vi "Lab_3.vi"() -> ()   [LabVIEW 2021]
panel:
  out "Real":dbl
  in  "Set_point":dbl
  out "k1":dbl[][](array[numeric])
  out "L":dbl[](array[numeric])
  out "p2":cdb
  out "p1":cdb
  out "p2_o":cdb
  out "p1_o":cdb
  in  "tso":dbl
  out "ks":dbl[][](array[numeric])
  out "Ki":dbl[][](array[numeric])
  out "K":dbl[](array[numeric])
  in  "T":dbl
  in  "tss":dbl
  in  "Fa":dbl
  in  "Orden":dbl
  out "Controlable":string="El sistema es Observable"
  out "Observable":string="El sistema es Observable"
  out "Waveform Chart 2":dbl[][](graph)
  out "Waveform Chart":dbl[][](graph)
  out "det_Mc":dbl
  out "det_Mo":dbl
  out "B_O":dbl[][](array[numeric])
  out "C_O":dbl[][](array[numeric])
  out "A_O":dbl[][](array[numeric])
  out "Rango_Con":dbl
  out "Rango_Obs":dbl
  out "C":dbl[][](array[numeric])
  out "B":dbl[][](array[numeric])
  out "A":dbl[][](array[numeric])
  out "Mo":dbl[][](array[numeric])
  out "Mc":dbl[][](array[numeric])
  in  "b4":dbl
  in  "b3":dbl
  in  "b2":dbl
  in  "b1":dbl
  in  "a4":dbl
  in  "a3":dbl
  in  "a2":dbl
  in  "a1":dbl
  # "Forma canónica observable (FCO)"
  # "Forma canónica controlable (FCC)"
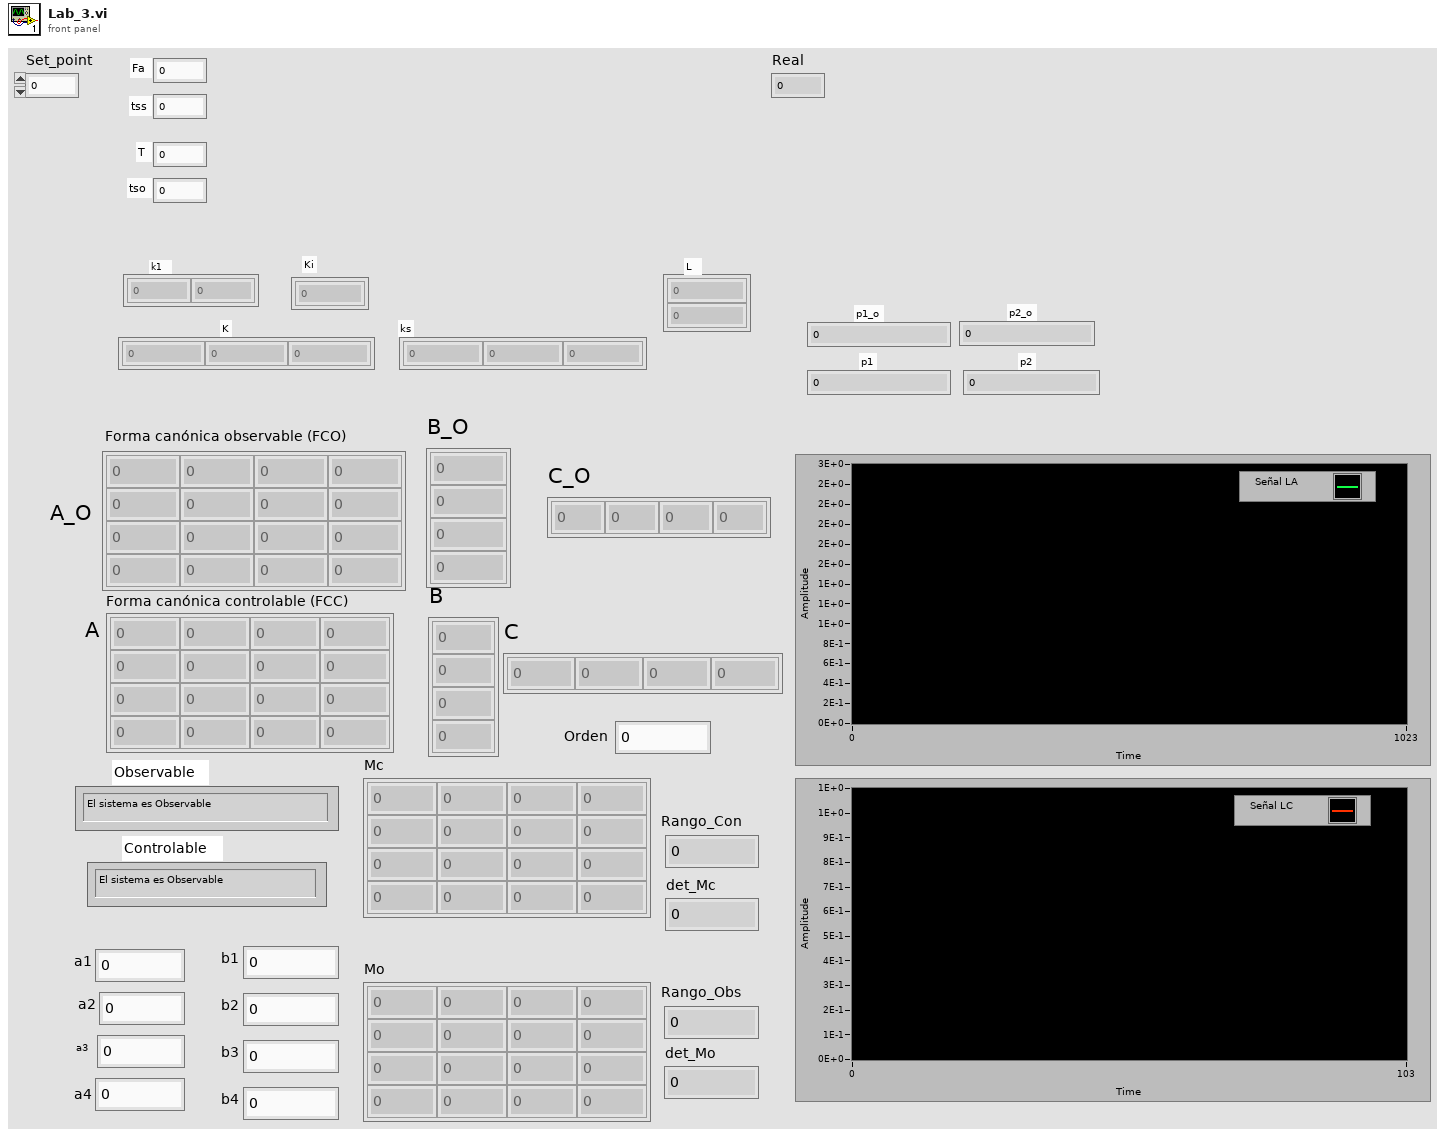
[diagram p1: front panel]
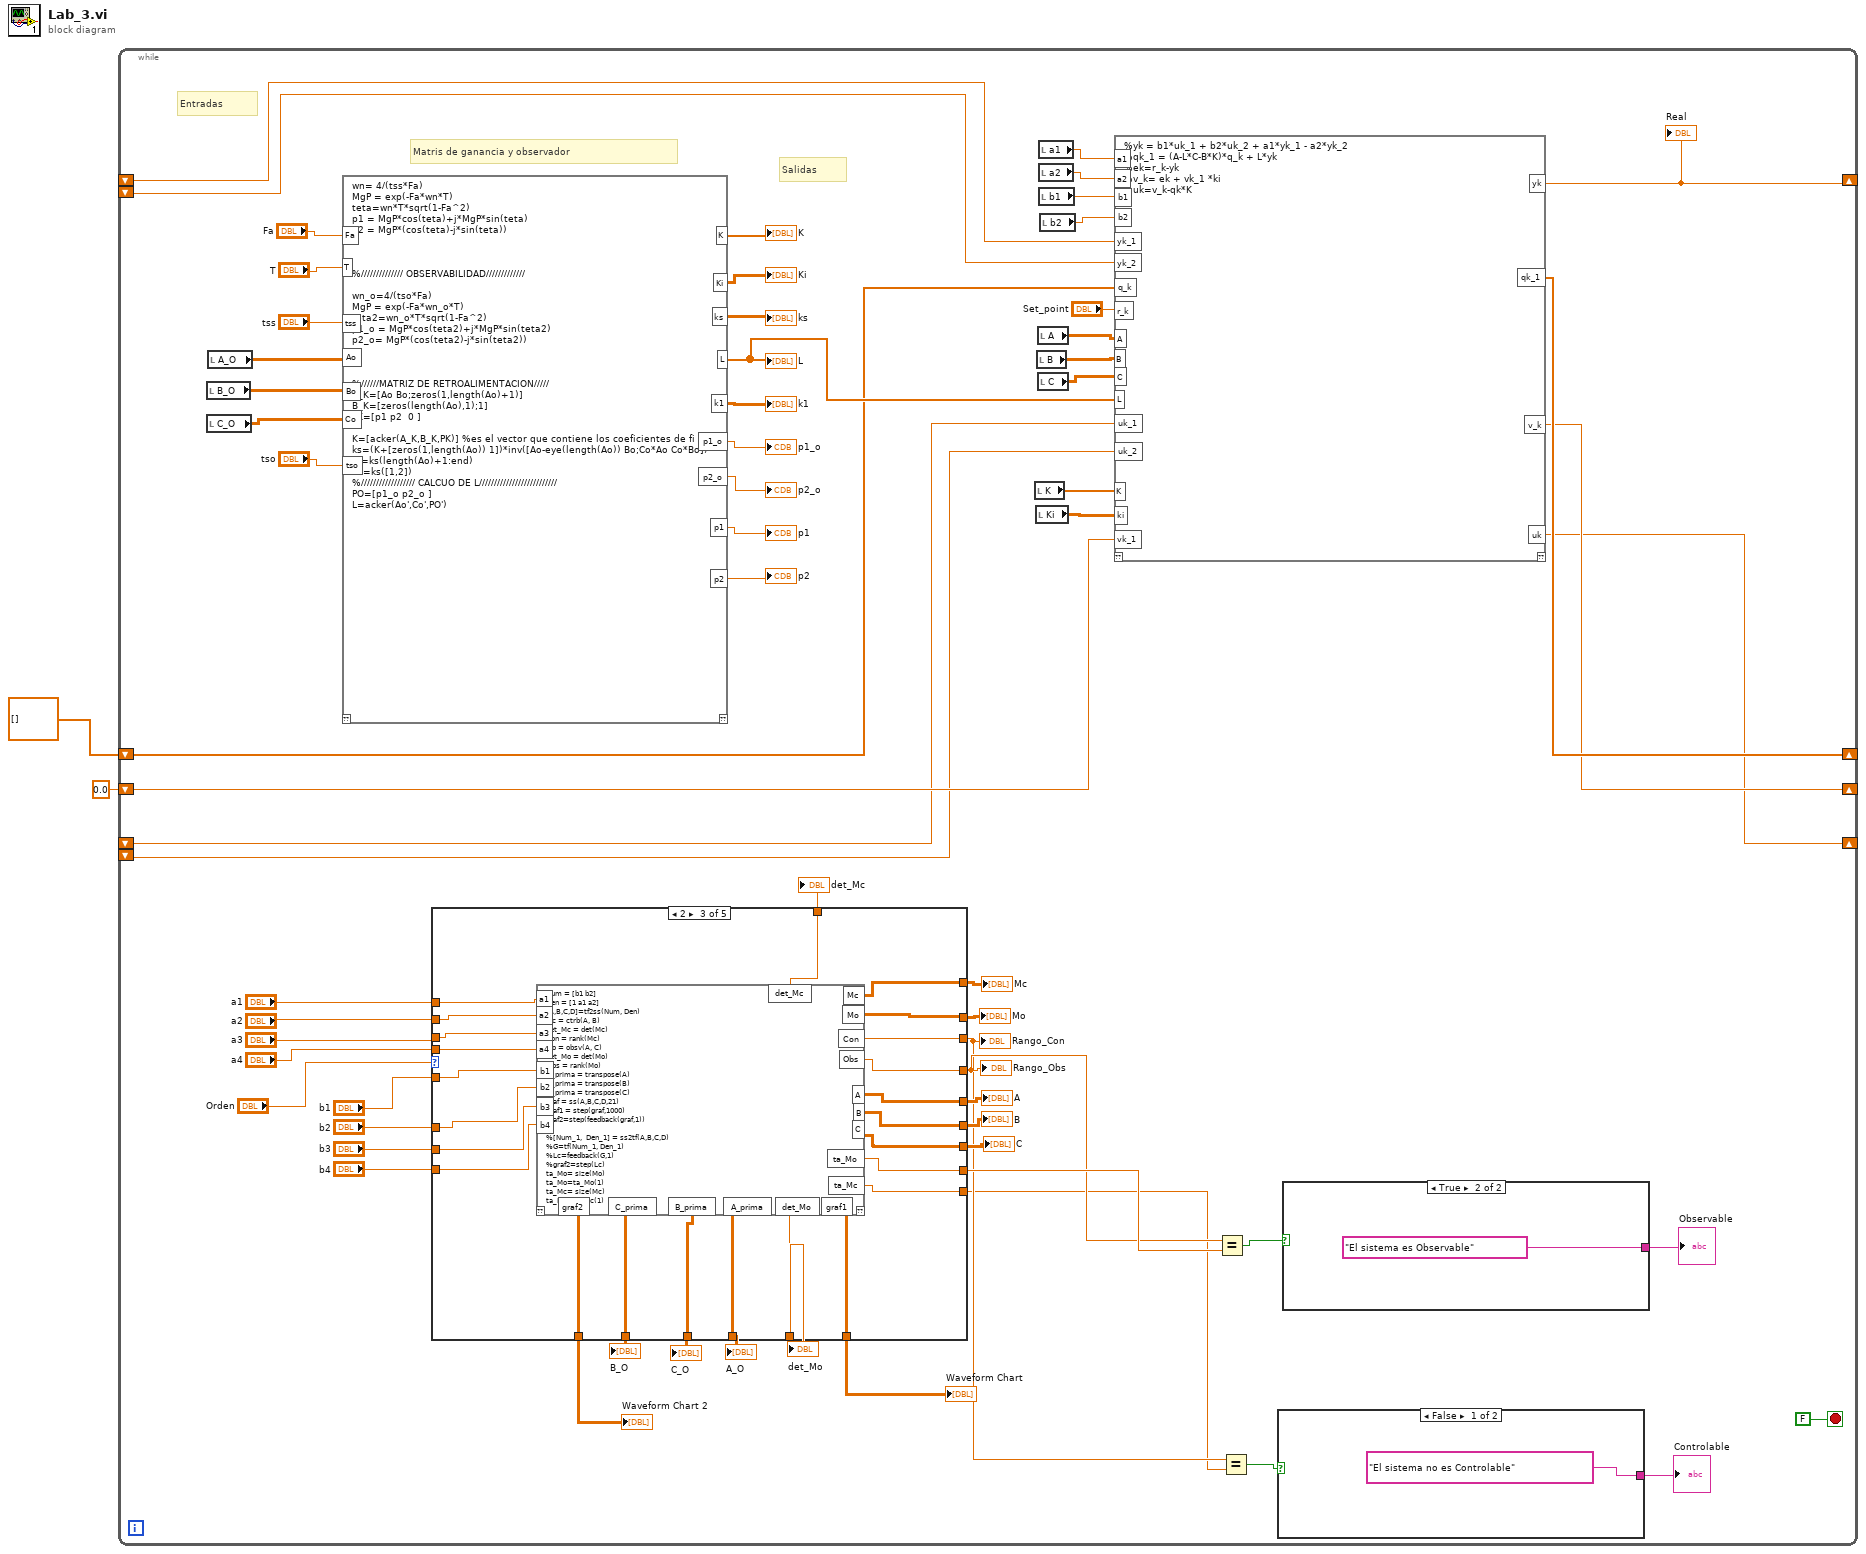
[diagram p0: block diagram]
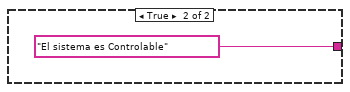
[diagram p2: hidden frame]
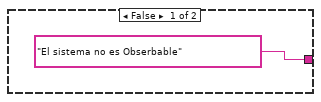
[diagram p3: hidden frame]
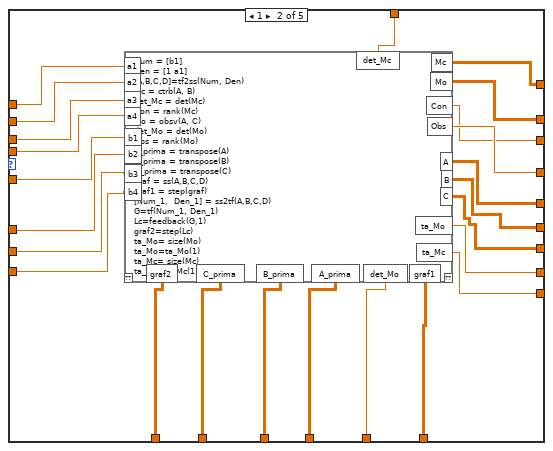
[diagram p5: hidden frame]
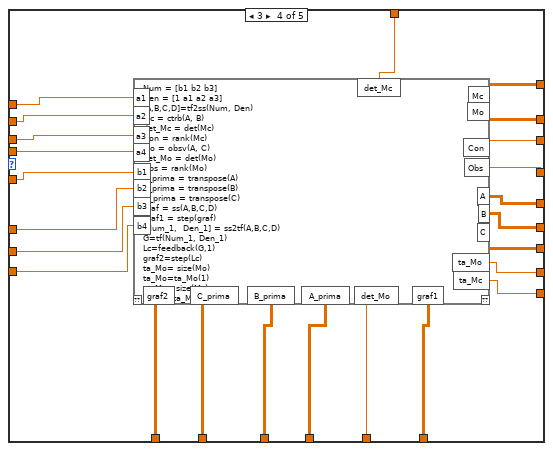
[diagram p6: hidden frame]
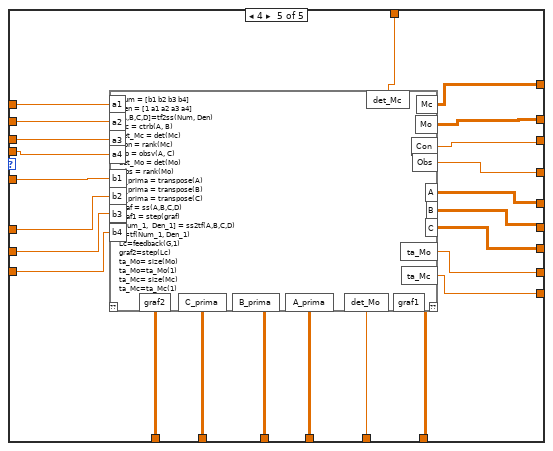
[diagram p7: hidden frame]
diagram:
  n1 = while {
    shift-right: [w14] -> _
    shift-left: _ -> [w16]
    shift-left: _ -> [w15]
    shift-right: [w12] -> _
    shift-left: dbl[] [] -> [w13]
    shift-right: [w10] -> _
    shift-left: 0.0 -> [w9]
    shift-right: [w5] -> _
    shift-left: _ -> [w4]
    shift-left: _ -> [w3]
    stop <- FALSE stop-if-true
    # "Matris de ganancia y observador"
    # "Salidas"
    # "Entradas"
    n2 = local read "B_O"() -> (w26:dbl[][])
    n3 = local read "C_O"() -> (w25:dbl[][])
    n4 = local read "A_O"() -> (w27:dbl[][])
    n5 = script code="wn= 4/(tss*Fa)\nMgP = exp(-Fa*wn*T)\nteta=wn*T*sqrt(1-Fa^2)\np1 = MgP*cos(teta)+j*MgP*sin(teta)\np2 = MgP*(cos(teta)-j*sin(teta))\n\n\n\n%////////////// OBSERVABILIDAD/////////////\n\nwn_o=4/(tso*Fa)\nMgP = exp(-Fa*wn_o*T)\nteta2=wn_o*T*sqrt(1-Fa^2)\np1_o = MgP*cos(teta2)+j*MgP*sin(teta2)\np2_o= MgP*(cos(teta2)-j*sin(teta2))\n\n\n\n%//////MATRIZ DE RETROALIMENTACION/////\nA_K=[Ao Bo;zeros(1,length(Ao)+1)]\nB_K=[zeros(length(Ao),1);1]\nPK=[p1 p2  0 ]\n\nK=[acker(A_K,B_K,PK)] %es el vector que contiene los coeficientes de fi de A\nks=(K+[zeros(1,length(Ao)) 1])*inv([Ao-eye(length(Ao)) Bo;Co*Ao Co*Bo])\nKi=ks(length(Ao)+1:end)\nk1=ks([1,2])\n%////////////////// CALCUO DE L//////////////////////////\nPO=[p1_o p2_o ]\nL=acker(Ao',Co',PO')"("Fa"="Fa", "T"="T", "tss"="tss", "Ao"=w27, "Bo"=w26, "Co"=w25, "tso"="tso") -> ("K"=→"K":dbl[], "Ki"=→"Ki":dbl[][], "ks"=→"ks":dbl[][], "L"=w21:dbl[], "k1"=→"k1":dbl[][], "p1_o"=→"p1_o":cdb, "p2_o"=→"p2_o":cdb, "p1"=→"p1":cdb, "p2"=→"p2":cdb)  [unwired: 1 in, 1 out]
    "L" <- w21
    n6 = case shown="2" "Orden" {
      tunnel: "b1" -> [_ w92 w116 w140 w168]
      tunnel: "b2" -> [_ w91 w115 w139 w167]
      tunnel: "b3" -> [_ w90 w114 w138 w166]
      tunnel: "b4" -> [_ w89 w113 w137 w165]
      tunnel: "a1" -> [_ w96 w120 w144 w164]
      tunnel: "a2" -> [_ w95 w119 w143 w163]
      tunnel: "a3" -> [_ w94 w118 w142 w162]
      tunnel: "a4" -> [_ w93 w117 w141 w161]
      tunnel: [_ w74 w112 w133 w157] -> w64
      tunnel: [_ w75 w111 w132 w156] -> w63
      tunnel: [_ w80 w110 w136 w158] -> w62
      tunnel: [_ w79 w109 w135 w159] -> w61
      tunnel: [_ w78 w108 w134 w160] -> w60
      tunnel: [_ w77 w107 w130 w154] -> w49
      tunnel: [_ w76 w106 w131 w155] -> w45
      tunnel: [_ w85 w105 w127 w153] -> w59
      tunnel: [_ w86 w104 w128 w152] -> w58
      tunnel: [_ w87 w103 w129 w151] -> w57
      tunnel: [_ w83 w102 w126 w150] -> w53
      tunnel: [_ w84 w100 w124 w149] -> w55
      tunnel: [_ w73 w101 w125 w148] -> w54
      tunnel: [_ w88 w99 w123 w147] -> w52
      tunnel: [_ w81 w98 w122 w146] -> w50
      tunnel: [_ w82 w97 w121 w145] -> w44
      frame 0, Default {
      }
      frame 1 {
        n7 = script code="Num = [b1]\nDen = [1 a1]\n[A,B,C,D]=tf2ss(Num, Den)\nMc = ctrb(A, B)\ndet_Mc = det(Mc)\nCon = rank(Mc)\nMo = obsv(A, C)\ndet_Mo = det(Mo)\nObs = rank(Mo)\nA_prima = transpose(A)\nB_prima = transpose(B)\nC_prima = transpose(C)\ngraf = ss(A,B,C,D)\ngraf1 = step(graf)\n[Num_1,  Den_1] = ss2tf(A,B,C,D)\nG=tf(Num_1, Den_1)\nLc=feedback(G,1)\ngraf2=step(Lc)\nta_Mo= size(Mo)\nta_Mo=ta_Mo(1)\nta_Mc= size(Mc)\nta_Mc=ta_Mc(1)"("b1"=w92, "b2"=w91, "b3"=w90, "b4"=w89, "a1"=w96, "a2"=w95, "a3"=w94, "a4"=w93) -> ("Mc"=w74:dbl[][], "Mo"=w75:dbl[][], "A"=w80:dbl[][], "B"=w79:dbl[][], "C"=w78:dbl[][], "Obs"=w77:dbl, "Con"=w76:dbl, "A_prima"=w85:dbl[][], "B_prima"=w86:dbl[][], "C_prima"=w87:dbl[][], "graf1"=w83:dbl[][], "det_Mc"=w73:dbl, "det_Mo"=w84:dbl, "graf2"=w88:dbl[][], "ta_Mo"=w81:dbl, "ta_Mc"=w82:dbl)  [unwired: 1 in, 1 out]
      }
      frame 2 {
        n8 = script code="Num = [b1 b2]\nDen = [1 a1 a2]\n[A,B,C,D]=tf2ss(Num, Den)\nMc = ctrb(A, B)\ndet_Mc = det(Mc)\nCon = rank(Mc)\nMo = obsv(A, C)\ndet_Mo = det(Mo)\nObs = rank(Mo)\nA_prima = transpose(A)\nB_prima = transpose(B)\nC_prima = transpose(C)\ngraf = ss(A,B,C,D,21)\ngraf1 = step(graf,1000)\ngraf2=step(feedback(graf,1))\n\n%[Num_1,  Den_1] = ss2tf(A,B,C,D)\n%G=tf(Num_1, Den_1)\n%Lc=feedback(G,1)\n%graf2=step(Lc)\nta_Mo= size(Mo)\nta_Mo=ta_Mo(1)\nta_Mc= size(Mc)\nta_Mc=ta_Mc(1)"("b1"=w116, "b2"=w115, "b3"=w114, "b4"=w113, "a1"=w120, "a2"=w119, "a3"=w118, "a4"=w117) -> ("Mc"=w112:dbl[][], "Mo"=w111:dbl[][], "A"=w110:dbl[][], "B"=w109:dbl[][], "C"=w108:dbl[][], "Obs"=w107:dbl, "Con"=w106:dbl, "A_prima"=w105:dbl[][], "B_prima"=w104:dbl[][], "C_prima"=w103:dbl[][], "graf1"=w102:dbl[][], "det_Mc"=w101:dbl, "det_Mo"=w100:dbl, "graf2"=w99:dbl[][], "ta_Mo"=w98:dbl, "ta_Mc"=w97:dbl)  [unwired: 1 in, 1 out]
      }
      frame 3 {
        n9 = script code="Num = [b1 b2 b3]\nDen = [1 a1 a2 a3]\n[A,B,C,D]=tf2ss(Num, Den)\nMc = ctrb(A, B)\ndet_Mc = det(Mc)\nCon = rank(Mc)\nMo = obsv(A, C)\ndet_Mo = det(Mo)\nObs = rank(Mo)\nA_prima = transpose(A)\nB_prima = transpose(B)\nC_prima = transpose(C)\ngraf = ss(A,B,C,D)\ngraf1 = step(graf)\n[Num_1,  Den_1] = ss2tf(A,B,C,D)\nG=tf(Num_1, Den_1)\nLc=feedback(G,1)\ngraf2=step(Lc)\nta_Mo= size(Mo)\nta_Mo=ta_Mo(1)\nta_Mc= size(Mc)\nta_Mc=ta_Mc(1)"("b1"=w140, "b2"=w139, "b3"=w138, "b4"=w137, "a1"=w144, "a2"=w143, "a3"=w142, "a4"=w141) -> ("Mc"=w133:dbl[][], "Mo"=w132:dbl[][], "A"=w136:dbl[][], "B"=w135:dbl[][], "C"=w134:dbl[][], "Con"=w131:dbl, "Obs"=w130:dbl, "A_prima"=w127:dbl[][], "B_prima"=w128:dbl[][], "C_prima"=w129:dbl[][], "graf1"=w126:dbl[][], "det_Mo"=w124:dbl, "det_Mc"=w125:dbl, "graf2"=w123:dbl[][], "ta_Mo"=w122:dbl, "ta_Mc"=w121:dbl)  [unwired: 1 in, 1 out]
      }
      frame 4 {
        n10 = script code="Num = [b1 b2 b3 b4]\nDen = [1 a1 a2 a3 a4]\n[A,B,C,D]=tf2ss(Num, Den)\nMc = ctrb(A, B)\ndet_Mc = det(Mc)\nCon = rank(Mc)\nMo = obsv(A, C)\ndet_Mo = det(Mo)\nObs = rank(Mo)\nA_prima = transpose(A)\nB_prima = transpose(B)\nC_prima = transpose(C)\ngraf = ss(A,B,C,D)\ngraf1 = step(graf)\n[Num_1,  Den_1] = ss2tf(A,B,C,D)\nG=tf(Num_1, Den_1)\nLc=feedback(G,1)\ngraf2=step(Lc)\nta_Mo= size(Mo)\nta_Mo=ta_Mo(1)\nta_Mc= size(Mc)\nta_Mc=ta_Mc(1)"("b1"=w168, "b2"=w167, "b3"=w166, "b4"=w165, "a1"=w164, "a2"=w163, "a3"=w162, "a4"=w161) -> ("Mc"=w157:dbl[][], "Mo"=w156:dbl[][], "A"=w158:dbl[][], "B"=w159:dbl[][], "C"=w160:dbl[][], "Con"=w155:dbl, "Obs"=w154:dbl, "A_prima"=w153:dbl[][], "B_prima"=w152:dbl[][], "C_prima"=w151:dbl[][], "graf1"=w150:dbl[][], "det_Mc"=w148:dbl, "det_Mo"=w149:dbl, "graf2"=w147:dbl[][], "ta_Mo"=w146:dbl, "ta_Mc"=w145:dbl)  [unwired: 1 in, 1 out]
      }
    }
    "Mc" <- w64
    "Mo" <- w63
    "A" <- w62
    "B" <- w61
    "C" <- w60
    "Rango_Obs" <- w49
    "Rango_Con" <- w45
    "A_O" <- w59
    "C_O" <- w58
    "B_O" <- w57
    "det_Mo" <- w55
    "det_Mc" <- w54
    "Waveform Chart" <- w53
    "Waveform Chart 2" <- w52
    n11 = local read "K"() -> (w6:dbl[])
    n12 = local read "Ki"() -> (w7:dbl[][])
    n13 = local read "B"() -> (w23:dbl[][])
    n14 = local read "A"() -> (w24:dbl[][])
    n15 = local read "C"() -> (w22:dbl[][])
    n16 = local read "a1"() -> (w20:dbl)
    n17 = local read "a2"() -> (w19:dbl)
    n18 = local read "b1"() -> (w18:dbl)
    n19 = local read "b2"() -> (w17:dbl)
    n20 = script code="%yk = b1*uk_1 + b2*uk_2 + a1*yk_1 - a2*yk_2\n%qk_1 = (A-L*C-B*K)*q_k + L*yk\n%ek=r_k-yk\n%v_k= ek + vk_1 *ki\n%uk=v_k-qk*K"("A"=w24, "L"=w21, "B"=w23, "C"=w22, "a1"=w20, "a2"=w19, "b1"=w18, "b2"=w17, "yk_1"=w16, "yk_2"=w15, "q_k"=w13, "r_k"="Set_point", "vk_1"=w9, "ki"=w7, "K"=w6, "uk_1"=w4, "uk_2"=w3) -> ("yk"=w14:dbl, "qk_1"=w12:dbl[], "v_k"=w10:dbl, "uk"=w5:dbl)  [unwired: 1 in, 1 out]
    "Real" <- w14
    n21 = Equal?(x=w49, y=w50) -> (x = y?=w48:bool)
    n22 = Equal?(x=w45, y=w44) -> (x = y?=w47:bool)
    n23 = case shown="False" w47 {
      tunnel: ["El sistema no es Controlable" "El sistema es Controlable"] -> w46
      frame False {
      }
      frame True {
      }
    }
    "Controlable" <- w46
    n24 = case shown="True" w48 {
      tunnel: ["El sistema no es Obserbable" "El sistema es Observable"] -> w51
      frame False {
      }
      frame True {
      }
    }
    "Observable" <- w51
  }
